vi "Convert String Block.vi"(0 "src buffer in":u8[](array[numeric]), 1 "dst buffer in":u8[](array[numeric]), 2 "src buffer offset":u64 format="%d bytes", 3 "dst buffer offset":u64 format="%d bytes", 4 "channel count":u64, 5 "error in (no error)":errorcluster, 6 "dst data type":T1, 8 "src data type":T1, 10 "dst byte order":T2(ring), 12 "src byte order":T2(ring)) -> (14 "src buffer out":u8[](array[numeric]), 15 "dst buffer out":u8[](array[numeric]), 19 "error out":errorcluster)   [LabVIEW 2017, in "String Type Converter.lvlib" / "String Type Converter.lvclass"]
uses:
  String Type Converter.lvclass
  Builds/Data Sharing Framework/Current/Core/DSF Core.lvlibp/Typedefs/DSF Data Type.ctl
  Builds/Data Sharing Framework/Current/Core/DSF Core.lvlibp/Classes/Framework/Framework.lvclass
  Builds/Data Sharing Framework/Current/Core/DSF Core.lvlibp
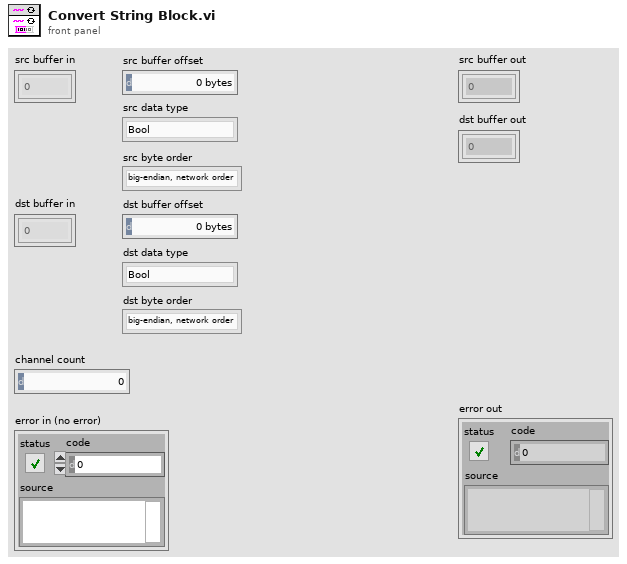
[diagram p1: front panel]
types:
  T1 = typedef "DSF Core.lvlibp/DSF Data Type.ctl" = enum8{"Bool", "SGL", "DBL", "I8", "I16", "I32", "I64", "U8", "U16", "U32", "U64"}
  T2 = enum16{"big-endian, network order", "native, host order", "little-endian"}
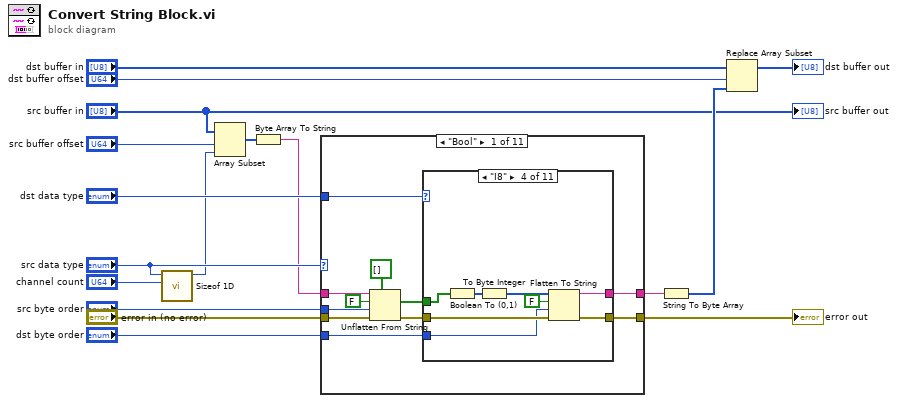
[diagram p0: block diagram]
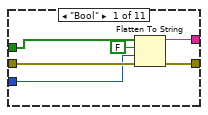
[diagram p2: hidden frame]
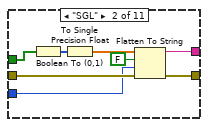
[diagram p3: hidden frame]
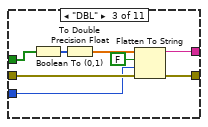
[diagram p4: hidden frame]
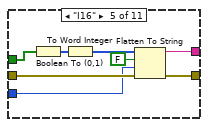
[diagram p5: hidden frame]
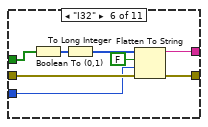
[diagram p6: hidden frame]
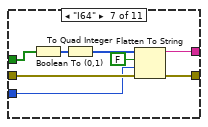
[diagram p7: hidden frame]
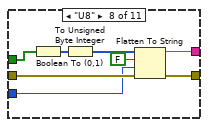
[diagram p8: hidden frame]
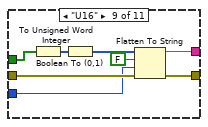
[diagram p9: hidden frame]
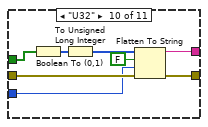
[diagram p10: hidden frame]
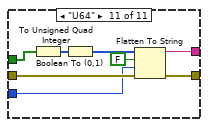
[diagram p11: hidden frame]
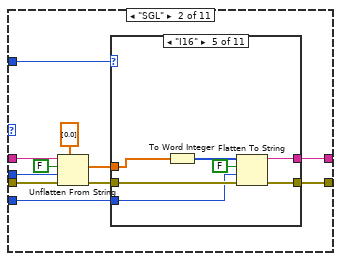
[diagram p12: hidden frame]
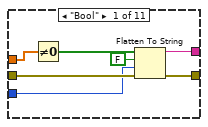
[diagram p13: hidden frame]
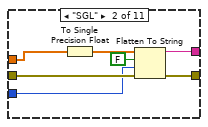
[diagram p14: hidden frame]
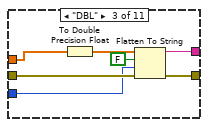
[diagram p15: hidden frame]
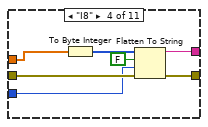
[diagram p16: hidden frame]
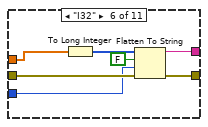
[diagram p17: hidden frame]
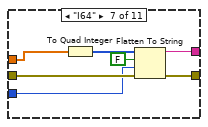
[diagram p18: hidden frame]
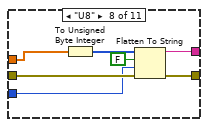
[diagram p19: hidden frame]
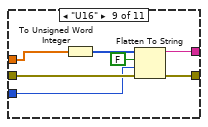
[diagram p20: hidden frame]
diagram:
  n1 = call "Sizeof 1D.vi"("count"="channel count", "data type"="src data type") -> ("size in bytes"=w3:u64)  [unwired: 9 in]
  n2 = Array Subset(array="src buffer in", index="src buffer offset", length=w3) -> (w2:u8[])
  n3 = Byte Array To String(unsigned byte array=w2) -> (string=w1:string)
  n4 = case shown="\"Bool\"" "src data type" {
    tunnel: w1 -> [w26 w123 w211 w299 w387 w475 w563 w651 w739 w827 w915]
    tunnel: "error in (no error)" -> [w25 w122 w210 w298 w386 w474 w562 w650 w738 w826 w914]
    tunnel: "dst data type" -> [w24 w121 w209 w297 w385 w473 w561 w649 w737 w825 w913]
    tunnel: [w21 w118 w206 w294 w382 w470 w558 w646 w734 w822 w910] -> w16
    tunnel: [w20 w117 w205 w293 w381 w469 w557 w645 w733 w821 w909] -> w10
    tunnel: "src byte order" -> [w19 w116 w204 w292 w380 w468 w556 w644 w732 w820 w908]
    tunnel: "dst byte order" -> [w18 w115 w203 w291 w379 w467 w555 w643 w731 w819 w907]
    frame "Bool" {
      n5 = Unflatten From String(type=bool[] [], binary string=w26, data includes array or string size? (T)=FALSE, byte order (0:big-endian, network order)=w19, error in (no error)=w25) -> (value=w23:bool[], error out=w22:errorcluster)  [unwired: 1 out]
      n6 = case shown="\"I8\"" w24 {
        tunnel: w23 -> [w34 w42 w50 w58 w66 w74 w82 w90 w98 w106 w114]
        tunnel: w22 -> [w33 w41 w49 w57 w65 w73 w81 w89 w97 w105 w113]
        tunnel: [w32 w40 w48 w56 w64 w72 w80 w88 w96 w104 w112] -> w21
        tunnel: [w31 w39 w47 w55 w63 w71 w79 w87 w95 w103 w111] -> w20
        tunnel: w18 -> [w30 w38 w46 w54 w62 w70 w78 w86 w94 w102 w110]
        frame "Bool" {
          n7 = Flatten To String(anything=w34, prepend array or string size? (T)=FALSE, byte order (0:big-endian, network order)=w30, error in (no error)=w33) -> (data string=w31:string, error out=w32:errorcluster)  [unwired: 1 out]
        }
        frame "SGL" {
          n8 = Boolean To (0,1)(Boolean=w42) -> (0, 1=w35:i16[])
          n9 = To Single Precision Float(number=w35) -> (single precision float=w36:sgl[])
          n10 = Flatten To String(anything=w36, prepend array or string size? (T)=FALSE, byte order (0:big-endian, network order)=w38, error in (no error)=w41) -> (data string=w39:string, error out=w40:errorcluster)  [unwired: 1 out]
        }
        frame "DBL" {
          n11 = Boolean To (0,1)(Boolean=w50) -> (0, 1=w43:i16[])
          n12 = To Double Precision Float(number=w43) -> (double precision float=w44:dbl[])
          n13 = Flatten To String(anything=w44, prepend array or string size? (T)=FALSE, byte order (0:big-endian, network order)=w46, error in (no error)=w49) -> (data string=w47:string, error out=w48:errorcluster)  [unwired: 1 out]
        }
        frame "I8" {
          n14 = Boolean To (0,1)(Boolean=w58) -> (0, 1=w51:i16[])
          n15 = To Byte Integer(number=w51) -> (8bit integer=w52:i8[])
          n16 = Flatten To String(anything=w52, prepend array or string size? (T)=FALSE, byte order (0:big-endian, network order)=w54, error in (no error)=w57) -> (data string=w55:string, error out=w56:errorcluster)  [unwired: 1 out]
        }
        frame "I16" {
          n17 = Boolean To (0,1)(Boolean=w66) -> (0, 1=w59:i16[])
          n18 = To Word Integer(number=w59) -> (16bit integer=w60:i16[])
          n19 = Flatten To String(anything=w60, prepend array or string size? (T)=FALSE, byte order (0:big-endian, network order)=w62, error in (no error)=w65) -> (data string=w63:string, error out=w64:errorcluster)  [unwired: 1 out]
        }
        frame "I32" {
          n20 = Boolean To (0,1)(Boolean=w74) -> (0, 1=w67:i16[])
          n21 = To Long Integer(number=w67) -> (32bit integer=w68:i32[])
          n22 = Flatten To String(anything=w68, prepend array or string size? (T)=FALSE, byte order (0:big-endian, network order)=w70, error in (no error)=w73) -> (data string=w71:string, error out=w72:errorcluster)  [unwired: 1 out]
        }
        frame "I64" {
          n23 = Boolean To (0,1)(Boolean=w82) -> (0, 1=w75:i16[])
          n24 = To Quad Integer(1:w75) -> (0:w76:i64[])
          n25 = Flatten To String(anything=w76, prepend array or string size? (T)=FALSE, byte order (0:big-endian, network order)=w78, error in (no error)=w81) -> (data string=w79:string, error out=w80:errorcluster)  [unwired: 1 out]
        }
        frame "U8" {
          n26 = Boolean To (0,1)(Boolean=w90) -> (0, 1=w83:i16[])
          n27 = To Unsigned Byte Integer(number=w83) -> (unsigned 8bit integer=w84:u8[])
          n28 = Flatten To String(anything=w84, prepend array or string size? (T)=FALSE, byte order (0:big-endian, network order)=w86, error in (no error)=w89) -> (data string=w87:string, error out=w88:errorcluster)  [unwired: 1 out]
        }
        frame "U16" {
          n29 = Boolean To (0,1)(Boolean=w98) -> (0, 1=w91:i16[])
          n30 = To Unsigned Word Integer(number=w91) -> (unsigned 16bit integer=w92:u16[])
          n31 = Flatten To String(anything=w92, prepend array or string size? (T)=FALSE, byte order (0:big-endian, network order)=w94, error in (no error)=w97) -> (data string=w95:string, error out=w96:errorcluster)  [unwired: 1 out]
        }
        frame "U32" {
          n32 = Boolean To (0,1)(Boolean=w106) -> (0, 1=w99:i16[])
          n33 = To Unsigned Long Integer(number=w99) -> (unsigned 32bit integer=w100:u32[])
          n34 = Flatten To String(anything=w100, prepend array or string size? (T)=FALSE, byte order (0:big-endian, network order)=w102, error in (no error)=w105) -> (data string=w103:string, error out=w104:errorcluster)  [unwired: 1 out]
        }
        frame "U64" {
          n35 = Boolean To (0,1)(Boolean=w114) -> (0, 1=w107:i16[])
          n36 = To Unsigned Quad Integer(1:w107) -> (0:w108:u64[])
          n37 = Flatten To String(anything=w108, prepend array or string size? (T)=FALSE, byte order (0:big-endian, network order)=w110, error in (no error)=w113) -> (data string=w111:string, error out=w112:errorcluster)  [unwired: 1 out]
        }
      }
    }
    frame "SGL" {
      n38 = Unflatten From String(type=sgl[] [0.0], binary string=w123, data includes array or string size? (T)=FALSE, byte order (0:big-endian, network order)=w116, error in (no error)=w122) -> (value=w120:sgl[], error out=w119:errorcluster)  [unwired: 1 out]
      n39 = case shown="\"I16\"" w121 {
        tunnel: w120 -> [w127 w134 w141 w148 w155 w162 w169 w176 w183 w190 w197]
        tunnel: w119 -> [w132 w139 w146 w153 w160 w167 w174 w181 w188 w195 w202]
        tunnel: [w131 w138 w145 w152 w159 w166 w173 w180 w187 w194 w201] -> w118
        tunnel: [w130 w137 w144 w151 w158 w165 w172 w179 w186 w193 w200] -> w117
        tunnel: w115 -> [w129 w136 w143 w150 w157 w164 w171 w178 w185 w192 w199]
        frame "Bool" {
          n40 = Not Equal To 0?(x=w127) -> (x != 0?=w126:bool[])
          n41 = Flatten To String(anything=w126, prepend array or string size? (T)=FALSE, byte order (0:big-endian, network order)=w129, error in (no error)=w132) -> (data string=w130:string, error out=w131:errorcluster)  [unwired: 1 out]
        }
        frame "SGL" {
          n42 = To Single Precision Float(number=w134) -> (single precision float=w133:sgl[])
          n43 = Flatten To String(anything=w133, prepend array or string size? (T)=FALSE, byte order (0:big-endian, network order)=w136, error in (no error)=w139) -> (data string=w137:string, error out=w138:errorcluster)  [unwired: 1 out]
        }
        frame "DBL" {
          n44 = To Double Precision Float(number=w141) -> (double precision float=w140:dbl[])
          n45 = Flatten To String(anything=w140, prepend array or string size? (T)=FALSE, byte order (0:big-endian, network order)=w143, error in (no error)=w146) -> (data string=w144:string, error out=w145:errorcluster)  [unwired: 1 out]
        }
        frame "I8" {
          n46 = To Byte Integer(number=w148) -> (8bit integer=w147:i8[])
          n47 = Flatten To String(anything=w147, prepend array or string size? (T)=FALSE, byte order (0:big-endian, network order)=w150, error in (no error)=w153) -> (data string=w151:string, error out=w152:errorcluster)  [unwired: 1 out]
        }
        frame "I16" {
          n48 = To Word Integer(number=w155) -> (16bit integer=w154:i16[])
          n49 = Flatten To String(anything=w154, prepend array or string size? (T)=FALSE, byte order (0:big-endian, network order)=w157, error in (no error)=w160) -> (data string=w158:string, error out=w159:errorcluster)  [unwired: 1 out]
        }
        frame "I32" {
          n50 = To Long Integer(number=w162) -> (32bit integer=w161:i32[])
          n51 = Flatten To String(anything=w161, prepend array or string size? (T)=FALSE, byte order (0:big-endian, network order)=w164, error in (no error)=w167) -> (data string=w165:string, error out=w166:errorcluster)  [unwired: 1 out]
        }
        frame "I64" {
          n52 = To Quad Integer(1:w169) -> (0:w168:i64[])
          n53 = Flatten To String(anything=w168, prepend array or string size? (T)=FALSE, byte order (0:big-endian, network order)=w171, error in (no error)=w174) -> (data string=w172:string, error out=w173:errorcluster)  [unwired: 1 out]
        }
        frame "U8" {
          n54 = To Unsigned Byte Integer(number=w176) -> (unsigned 8bit integer=w175:u8[])
          n55 = Flatten To String(anything=w175, prepend array or string size? (T)=FALSE, byte order (0:big-endian, network order)=w178, error in (no error)=w181) -> (data string=w179:string, error out=w180:errorcluster)  [unwired: 1 out]
        }
        frame "U16" {
          n56 = To Unsigned Word Integer(number=w183) -> (unsigned 16bit integer=w182:u16[])
          n57 = Flatten To String(anything=w182, prepend array or string size? (T)=FALSE, byte order (0:big-endian, network order)=w185, error in (no error)=w188) -> (data string=w186:string, error out=w187:errorcluster)  [unwired: 1 out]
        }
        frame "U32" {
          n58 = To Unsigned Long Integer(number=w190) -> (unsigned 32bit integer=w189:u32[])
          n59 = Flatten To String(anything=w189, prepend array or string size? (T)=FALSE, byte order (0:big-endian, network order)=w192, error in (no error)=w195) -> (data string=w193:string, error out=w194:errorcluster)  [unwired: 1 out]
        }
        frame "U64" {
          n60 = To Unsigned Quad Integer(1:w197) -> (0:w196:u64[])
          n61 = Flatten To String(anything=w196, prepend array or string size? (T)=FALSE, byte order (0:big-endian, network order)=w199, error in (no error)=w202) -> (data string=w200:string, error out=w201:errorcluster)  [unwired: 1 out]
        }
      }
    }
    frame "DBL" {
      n62 = Unflatten From String(type=dbl[] [0.0], binary string=w211, data includes array or string size? (T)=FALSE, byte order (0:big-endian, network order)=w204, error in (no error)=w210) -> (value=w208:dbl[], error out=w207:errorcluster)  [unwired: 1 out]
      n63 = case shown="\"U64\"" w209 {
        tunnel: w208 -> [w215 w222 w229 w236 w243 w250 w257 w264 w271 w278 w285]
        tunnel: w207 -> [w220 w227 w234 w241 w248 w255 w262 w269 w276 w283 w290]
        tunnel: [w219 w226 w233 w240 w247 w254 w261 w268 w275 w282 w289] -> w206
        tunnel: [w218 w225 w232 w239 w246 w253 w260 w267 w274 w281 w288] -> w205
        tunnel: w203 -> [w217 w224 w231 w238 w245 w252 w259 w266 w273 w280 w287]
        frame "Bool" {
          n64 = Not Equal To 0?(x=w215) -> (x != 0?=w214:bool[])
          n65 = Flatten To String(anything=w214, prepend array or string size? (T)=FALSE, byte order (0:big-endian, network order)=w217, error in (no error)=w220) -> (data string=w218:string, error out=w219:errorcluster)  [unwired: 1 out]
        }
        frame "SGL" {
          n66 = To Single Precision Float(number=w222) -> (single precision float=w221:sgl[])
          n67 = Flatten To String(anything=w221, prepend array or string size? (T)=FALSE, byte order (0:big-endian, network order)=w224, error in (no error)=w227) -> (data string=w225:string, error out=w226:errorcluster)  [unwired: 1 out]
        }
        frame "DBL" {
          n68 = To Double Precision Float(number=w229) -> (double precision float=w228:dbl[])
          n69 = Flatten To String(anything=w228, prepend array or string size? (T)=FALSE, byte order (0:big-endian, network order)=w231, error in (no error)=w234) -> (data string=w232:string, error out=w233:errorcluster)  [unwired: 1 out]
        }
        frame "I8" {
          n70 = To Byte Integer(number=w236) -> (8bit integer=w235:i8[])
          n71 = Flatten To String(anything=w235, prepend array or string size? (T)=FALSE, byte order (0:big-endian, network order)=w238, error in (no error)=w241) -> (data string=w239:string, error out=w240:errorcluster)  [unwired: 1 out]
        }
        frame "I16" {
          n72 = To Word Integer(number=w243) -> (16bit integer=w242:i16[])
          n73 = Flatten To String(anything=w242, prepend array or string size? (T)=FALSE, byte order (0:big-endian, network order)=w245, error in (no error)=w248) -> (data string=w246:string, error out=w247:errorcluster)  [unwired: 1 out]
        }
        frame "I32" {
          n74 = To Long Integer(number=w250) -> (32bit integer=w249:i32[])
          n75 = Flatten To String(anything=w249, prepend array or string size? (T)=FALSE, byte order (0:big-endian, network order)=w252, error in (no error)=w255) -> (data string=w253:string, error out=w254:errorcluster)  [unwired: 1 out]
        }
        frame "I64" {
          n76 = To Quad Integer(1:w257) -> (0:w256:i64[])
          n77 = Flatten To String(anything=w256, prepend array or string size? (T)=FALSE, byte order (0:big-endian, network order)=w259, error in (no error)=w262) -> (data string=w260:string, error out=w261:errorcluster)  [unwired: 1 out]
        }
        frame "U8" {
          n78 = To Unsigned Byte Integer(number=w264) -> (unsigned 8bit integer=w263:u8[])
          n79 = Flatten To String(anything=w263, prepend array or string size? (T)=FALSE, byte order (0:big-endian, network order)=w266, error in (no error)=w269) -> (data string=w267:string, error out=w268:errorcluster)  [unwired: 1 out]
        }
        frame "U16" {
          n80 = To Unsigned Word Integer(number=w271) -> (unsigned 16bit integer=w270:u16[])
          n81 = Flatten To String(anything=w270, prepend array or string size? (T)=FALSE, byte order (0:big-endian, network order)=w273, error in (no error)=w276) -> (data string=w274:string, error out=w275:errorcluster)  [unwired: 1 out]
        }
        frame "U32" {
          n82 = To Unsigned Long Integer(number=w278) -> (unsigned 32bit integer=w277:u32[])
          n83 = Flatten To String(anything=w277, prepend array or string size? (T)=FALSE, byte order (0:big-endian, network order)=w280, error in (no error)=w283) -> (data string=w281:string, error out=w282:errorcluster)  [unwired: 1 out]
        }
        frame "U64" {
          n84 = To Unsigned Quad Integer(1:w285) -> (0:w284:u64[])
          n85 = Flatten To String(anything=w284, prepend array or string size? (T)=FALSE, byte order (0:big-endian, network order)=w287, error in (no error)=w290) -> (data string=w288:string, error out=w289:errorcluster)  [unwired: 1 out]
        }
      }
    }
    frame "I8" {
      n86 = Unflatten From String(type=i8[] [0], binary string=w299, data includes array or string size? (T)=FALSE, byte order (0:big-endian, network order)=w292, error in (no error)=w298) -> (value=w296:i8[], error out=w295:errorcluster)  [unwired: 1 out]
      n87 = case shown="\"Bool\"" w297 {
        tunnel: w296 -> [w303 w310 w317 w324 w331 w338 w345 w352 w359 w366 w373]
        tunnel: w295 -> [w308 w315 w322 w329 w336 w343 w350 w357 w364 w371 w378]
        tunnel: [w307 w314 w321 w328 w335 w342 w349 w356 w363 w370 w377] -> w294
        tunnel: [w306 w313 w320 w327 w334 w341 w348 w355 w362 w369 w376] -> w293
        tunnel: w291 -> [w305 w312 w319 w326 w333 w340 w347 w354 w361 w368 w375]
        frame "Bool" {
          n88 = Not Equal To 0?(x=w303) -> (x != 0?=w302:bool[])
          n89 = Flatten To String(anything=w302, prepend array or string size? (T)=FALSE, byte order (0:big-endian, network order)=w305, error in (no error)=w308) -> (data string=w306:string, error out=w307:errorcluster)  [unwired: 1 out]
        }
        frame "SGL" {
          n90 = To Single Precision Float(number=w310) -> (single precision float=w309:sgl[])
          n91 = Flatten To String(anything=w309, prepend array or string size? (T)=FALSE, byte order (0:big-endian, network order)=w312, error in (no error)=w315) -> (data string=w313:string, error out=w314:errorcluster)  [unwired: 1 out]
        }
        frame "DBL" {
          n92 = To Double Precision Float(number=w317) -> (double precision float=w316:dbl[])
          n93 = Flatten To String(anything=w316, prepend array or string size? (T)=FALSE, byte order (0:big-endian, network order)=w319, error in (no error)=w322) -> (data string=w320:string, error out=w321:errorcluster)  [unwired: 1 out]
        }
        frame "I8" {
          n94 = To Byte Integer(number=w324) -> (8bit integer=w323:i8[])
          n95 = Flatten To String(anything=w323, prepend array or string size? (T)=FALSE, byte order (0:big-endian, network order)=w326, error in (no error)=w329) -> (data string=w327:string, error out=w328:errorcluster)  [unwired: 1 out]
        }
        frame "I16" {
          n96 = To Word Integer(number=w331) -> (16bit integer=w330:i16[])
          n97 = Flatten To String(anything=w330, prepend array or string size? (T)=FALSE, byte order (0:big-endian, network order)=w333, error in (no error)=w336) -> (data string=w334:string, error out=w335:errorcluster)  [unwired: 1 out]
        }
        frame "I32" {
          n98 = To Long Integer(number=w338) -> (32bit integer=w337:i32[])
          n99 = Flatten To String(anything=w337, prepend array or string size? (T)=FALSE, byte order (0:big-endian, network order)=w340, error in (no error)=w343) -> (data string=w341:string, error out=w342:errorcluster)  [unwired: 1 out]
        }
        frame "I64" {
          n100 = To Quad Integer(1:w345) -> (0:w344:i64[])
          n101 = Flatten To String(anything=w344, prepend array or string size? (T)=FALSE, byte order (0:big-endian, network order)=w347, error in (no error)=w350) -> (data string=w348:string, error out=w349:errorcluster)  [unwired: 1 out]
        }
        frame "U8" {
          n102 = To Unsigned Byte Integer(number=w352) -> (unsigned 8bit integer=w351:u8[])
          n103 = Flatten To String(anything=w351, prepend array or string size? (T)=FALSE, byte order (0:big-endian, network order)=w354, error in (no error)=w357) -> (data string=w355:string, error out=w356:errorcluster)  [unwired: 1 out]
        }
        frame "U16" {
          n104 = To Unsigned Word Integer(number=w359) -> (unsigned 16bit integer=w358:u16[])
          n105 = Flatten To String(anything=w358, prepend array or string size? (T)=FALSE, byte order (0:big-endian, network order)=w361, error in (no error)=w364) -> (data string=w362:string, error out=w363:errorcluster)  [unwired: 1 out]
        }
        frame "U32" {
          n106 = To Unsigned Long Integer(number=w366) -> (unsigned 32bit integer=w365:u32[])
          n107 = Flatten To String(anything=w365, prepend array or string size? (T)=FALSE, byte order (0:big-endian, network order)=w368, error in (no error)=w371) -> (data string=w369:string, error out=w370:errorcluster)  [unwired: 1 out]
        }
        frame "U64" {
          n108 = To Unsigned Quad Integer(1:w373) -> (0:w372:u64[])
          n109 = Flatten To String(anything=w372, prepend array or string size? (T)=FALSE, byte order (0:big-endian, network order)=w375, error in (no error)=w378) -> (data string=w376:string, error out=w377:errorcluster)  [unwired: 1 out]
        }
      }
    }
    frame "I16" {
      n110 = Unflatten From String(type=i16[] [0], binary string=w387, data includes array or string size? (T)=FALSE, byte order (0:big-endian, network order)=w380, error in (no error)=w386) -> (value=w384:i16[], error out=w383:errorcluster)  [unwired: 1 out]
      n111 = case shown="\"Bool\"" w385 {
        tunnel: w384 -> [w391 w398 w405 w412 w419 w426 w433 w440 w447 w454 w461]
        tunnel: w383 -> [w396 w403 w410 w417 w424 w431 w438 w445 w452 w459 w466]
        tunnel: [w395 w402 w409 w416 w423 w430 w437 w444 w451 w458 w465] -> w382
        tunnel: [w394 w401 w408 w415 w422 w429 w436 w443 w450 w457 w464] -> w381
        tunnel: w379 -> [w393 w400 w407 w414 w421 w428 w435 w442 w449 w456 w463]
        frame "Bool" {
          n112 = Not Equal To 0?(x=w391) -> (x != 0?=w390:bool[])
          n113 = Flatten To String(anything=w390, prepend array or string size? (T)=FALSE, byte order (0:big-endian, network order)=w393, error in (no error)=w396) -> (data string=w394:string, error out=w395:errorcluster)  [unwired: 1 out]
        }
        frame "SGL" {
          n114 = To Single Precision Float(number=w398) -> (single precision float=w397:sgl[])
          n115 = Flatten To String(anything=w397, prepend array or string size? (T)=FALSE, byte order (0:big-endian, network order)=w400, error in (no error)=w403) -> (data string=w401:string, error out=w402:errorcluster)  [unwired: 1 out]
        }
        frame "DBL" {
          n116 = To Double Precision Float(number=w405) -> (double precision float=w404:dbl[])
          n117 = Flatten To String(anything=w404, prepend array or string size? (T)=FALSE, byte order (0:big-endian, network order)=w407, error in (no error)=w410) -> (data string=w408:string, error out=w409:errorcluster)  [unwired: 1 out]
        }
        frame "I8" {
          n118 = To Byte Integer(number=w412) -> (8bit integer=w411:i8[])
          n119 = Flatten To String(anything=w411, prepend array or string size? (T)=FALSE, byte order (0:big-endian, network order)=w414, error in (no error)=w417) -> (data string=w415:string, error out=w416:errorcluster)  [unwired: 1 out]
        }
        frame "I16" {
          n120 = To Word Integer(number=w419) -> (16bit integer=w418:i16[])
          n121 = Flatten To String(anything=w418, prepend array or string size? (T)=FALSE, byte order (0:big-endian, network order)=w421, error in (no error)=w424) -> (data string=w422:string, error out=w423:errorcluster)  [unwired: 1 out]
        }
        frame "I32" {
          n122 = To Long Integer(number=w426) -> (32bit integer=w425:i32[])
          n123 = Flatten To String(anything=w425, prepend array or string size? (T)=FALSE, byte order (0:big-endian, network order)=w428, error in (no error)=w431) -> (data string=w429:string, error out=w430:errorcluster)  [unwired: 1 out]
        }
        frame "I64" {
          n124 = To Quad Integer(1:w433) -> (0:w432:i64[])
          n125 = Flatten To String(anything=w432, prepend array or string size? (T)=FALSE, byte order (0:big-endian, network order)=w435, error in (no error)=w438) -> (data string=w436:string, error out=w437:errorcluster)  [unwired: 1 out]
        }
        frame "U8" {
          n126 = To Unsigned Byte Integer(number=w440) -> (unsigned 8bit integer=w439:u8[])
          n127 = Flatten To String(anything=w439, prepend array or string size? (T)=FALSE, byte order (0:big-endian, network order)=w442, error in (no error)=w445) -> (data string=w443:string, error out=w444:errorcluster)  [unwired: 1 out]
        }
        frame "U16" {
          n128 = To Unsigned Word Integer(number=w447) -> (unsigned 16bit integer=w446:u16[])
          n129 = Flatten To String(anything=w446, prepend array or string size? (T)=FALSE, byte order (0:big-endian, network order)=w449, error in (no error)=w452) -> (data string=w450:string, error out=w451:errorcluster)  [unwired: 1 out]
        }
        frame "U32" {
          n130 = To Unsigned Long Integer(number=w454) -> (unsigned 32bit integer=w453:u32[])
          n131 = Flatten To String(anything=w453, prepend array or string size? (T)=FALSE, byte order (0:big-endian, network order)=w456, error in (no error)=w459) -> (data string=w457:string, error out=w458:errorcluster)  [unwired: 1 out]
        }
        frame "U64" {
          n132 = To Unsigned Quad Integer(1:w461) -> (0:w460:u64[])
          n133 = Flatten To String(anything=w460, prepend array or string size? (T)=FALSE, byte order (0:big-endian, network order)=w463, error in (no error)=w466) -> (data string=w464:string, error out=w465:errorcluster)  [unwired: 1 out]
        }
      }
    }
    frame "I32" {
      n134 = Unflatten From String(type=i32[] [0], binary string=w475, data includes array or string size? (T)=FALSE, byte order (0:big-endian, network order)=w468, error in (no error)=w474) -> (value=w472:i32[], error out=w471:errorcluster)  [unwired: 1 out]
      n135 = case shown="\"Bool\"" w473 {
        tunnel: w472 -> [w479 w486 w493 w500 w507 w514 w521 w528 w535 w542 w549]
        tunnel: w471 -> [w484 w491 w498 w505 w512 w519 w526 w533 w540 w547 w554]
        tunnel: [w483 w490 w497 w504 w511 w518 w525 w532 w539 w546 w553] -> w470
        tunnel: [w482 w489 w496 w503 w510 w517 w524 w531 w538 w545 w552] -> w469
        tunnel: w467 -> [w481 w488 w495 w502 w509 w516 w523 w530 w537 w544 w551]
        frame "Bool" {
          n136 = Not Equal To 0?(x=w479) -> (x != 0?=w478:bool[])
          n137 = Flatten To String(anything=w478, prepend array or string size? (T)=FALSE, byte order (0:big-endian, network order)=w481, error in (no error)=w484) -> (data string=w482:string, error out=w483:errorcluster)  [unwired: 1 out]
        }
        frame "SGL" {
          n138 = To Single Precision Float(number=w486) -> (single precision float=w485:sgl[])
          n139 = Flatten To String(anything=w485, prepend array or string size? (T)=FALSE, byte order (0:big-endian, network order)=w488, error in (no error)=w491) -> (data string=w489:string, error out=w490:errorcluster)  [unwired: 1 out]
        }
        frame "DBL" {
          n140 = To Double Precision Float(number=w493) -> (double precision float=w492:dbl[])
          n141 = Flatten To String(anything=w492, prepend array or string size? (T)=FALSE, byte order (0:big-endian, network order)=w495, error in (no error)=w498) -> (data string=w496:string, error out=w497:errorcluster)  [unwired: 1 out]
        }
        frame "I8" {
          n142 = To Byte Integer(number=w500) -> (8bit integer=w499:i8[])
          n143 = Flatten To String(anything=w499, prepend array or string size? (T)=FALSE, byte order (0:big-endian, network order)=w502, error in (no error)=w505) -> (data string=w503:string, error out=w504:errorcluster)  [unwired: 1 out]
        }
        frame "I16" {
          n144 = To Word Integer(number=w507) -> (16bit integer=w506:i16[])
          n145 = Flatten To String(anything=w506, prepend array or string size? (T)=FALSE, byte order (0:big-endian, network order)=w509, error in (no error)=w512) -> (data string=w510:string, error out=w511:errorcluster)  [unwired: 1 out]
        }
        frame "I32" {
          n146 = To Long Integer(number=w514) -> (32bit integer=w513:i32[])
          n147 = Flatten To String(anything=w513, prepend array or string size? (T)=FALSE, byte order (0:big-endian, network order)=w516, error in (no error)=w519) -> (data string=w517:string, error out=w518:errorcluster)  [unwired: 1 out]
        }
        frame "I64" {
          n148 = To Quad Integer(1:w521) -> (0:w520:i64[])
          n149 = Flatten To String(anything=w520, prepend array or string size? (T)=FALSE, byte order (0:big-endian, network order)=w523, error in (no error)=w526) -> (data string=w524:string, error out=w525:errorcluster)  [unwired: 1 out]
        }
        frame "U8" {
          n150 = To Unsigned Byte Integer(number=w528) -> (unsigned 8bit integer=w527:u8[])
          n151 = Flatten To String(anything=w527, prepend array or string size? (T)=FALSE, byte order (0:big-endian, network order)=w530, error in (no error)=w533) -> (data string=w531:string, error out=w532:errorcluster)  [unwired: 1 out]
        }
        frame "U16" {
          n152 = To Unsigned Word Integer(number=w535) -> (unsigned 16bit integer=w534:u16[])
          n153 = Flatten To String(anything=w534, prepend array or string size? (T)=FALSE, byte order (0:big-endian, network order)=w537, error in (no error)=w540) -> (data string=w538:string, error out=w539:errorcluster)  [unwired: 1 out]
        }
        frame "U32" {
          n154 = To Unsigned Long Integer(number=w542) -> (unsigned 32bit integer=w541:u32[])
          n155 = Flatten To String(anything=w541, prepend array or string size? (T)=FALSE, byte order (0:big-endian, network order)=w544, error in (no error)=w547) -> (data string=w545:string, error out=w546:errorcluster)  [unwired: 1 out]
        }
        frame "U64" {
          n156 = To Unsigned Quad Integer(1:w549) -> (0:w548:u64[])
          n157 = Flatten To String(anything=w548, prepend array or string size? (T)=FALSE, byte order (0:big-endian, network order)=w551, error in (no error)=w554) -> (data string=w552:string, error out=w553:errorcluster)  [unwired: 1 out]
        }
      }
    }
    frame "I64" {
      n158 = Unflatten From String(type=i64[] [0], binary string=w563, data includes array or string size? (T)=FALSE, byte order (0:big-endian, network order)=w556, error in (no error)=w562) -> (value=w560:i64[], error out=w559:errorcluster)  [unwired: 1 out]
      n159 = case shown="\"Bool\"" w561 {
        tunnel: w560 -> [w567 w574 w581 w588 w595 w602 w609 w616 w623 w630 w637]
        tunnel: w559 -> [w572 w579 w586 w593 w600 w607 w614 w621 w628 w635 w642]
        tunnel: [w571 w578 w585 w592 w599 w606 w613 w620 w627 w634 w641] -> w558
        tunnel: [w570 w577 w584 w591 w598 w605 w612 w619 w626 w633 w640] -> w557
        tunnel: w555 -> [w569 w576 w583 w590 w597 w604 w611 w618 w625 w632 w639]
        frame "Bool" {
          n160 = Not Equal To 0?(x=w567) -> (x != 0?=w566:bool[])
          n161 = Flatten To String(anything=w566, prepend array or string size? (T)=FALSE, byte order (0:big-endian, network order)=w569, error in (no error)=w572) -> (data string=w570:string, error out=w571:errorcluster)  [unwired: 1 out]
        }
        frame "SGL" {
          n162 = To Single Precision Float(number=w574) -> (single precision float=w573:sgl[])
          n163 = Flatten To String(anything=w573, prepend array or string size? (T)=FALSE, byte order (0:big-endian, network order)=w576, error in (no error)=w579) -> (data string=w577:string, error out=w578:errorcluster)  [unwired: 1 out]
        }
        frame "DBL" {
          n164 = To Double Precision Float(number=w581) -> (double precision float=w580:dbl[])
          n165 = Flatten To String(anything=w580, prepend array or string size? (T)=FALSE, byte order (0:big-endian, network order)=w583, error in (no error)=w586) -> (data string=w584:string, error out=w585:errorcluster)  [unwired: 1 out]
        }
        frame "I8" {
          n166 = To Byte Integer(number=w588) -> (8bit integer=w587:i8[])
          n167 = Flatten To String(anything=w587, prepend array or string size? (T)=FALSE, byte order (0:big-endian, network order)=w590, error in (no error)=w593) -> (data string=w591:string, error out=w592:errorcluster)  [unwired: 1 out]
        }
        frame "I16" {
          n168 = To Word Integer(number=w595) -> (16bit integer=w594:i16[])
          n169 = Flatten To String(anything=w594, prepend array or string size? (T)=FALSE, byte order (0:big-endian, network order)=w597, error in (no error)=w600) -> (data string=w598:string, error out=w599:errorcluster)  [unwired: 1 out]
        }
        frame "I32" {
          n170 = To Long Integer(number=w602) -> (32bit integer=w601:i32[])
          n171 = Flatten To String(anything=w601, prepend array or string size? (T)=FALSE, byte order (0:big-endian, network order)=w604, error in (no error)=w607) -> (data string=w605:string, error out=w606:errorcluster)  [unwired: 1 out]
        }
        frame "I64" {
          n172 = To Quad Integer(1:w609) -> (0:w608:i64[])
          n173 = Flatten To String(anything=w608, prepend array or string size? (T)=FALSE, byte order (0:big-endian, network order)=w611, error in (no error)=w614) -> (data string=w612:string, error out=w613:errorcluster)  [unwired: 1 out]
        }
        frame "U8" {
          n174 = To Unsigned Byte Integer(number=w616) -> (unsigned 8bit integer=w615:u8[])
          n175 = Flatten To String(anything=w615, prepend array or string size? (T)=FALSE, byte order (0:big-endian, network order)=w618, error in (no error)=w621) -> (data string=w619:string, error out=w620:errorcluster)  [unwired: 1 out]
        }
        frame "U16" {
          n176 = To Unsigned Word Integer(number=w623) -> (unsigned 16bit integer=w622:u16[])
          n177 = Flatten To String(anything=w622, prepend array or string size? (T)=FALSE, byte order (0:big-endian, network order)=w625, error in (no error)=w628) -> (data string=w626:string, error out=w627:errorcluster)  [unwired: 1 out]
        }
        frame "U32" {
          n178 = To Unsigned Long Integer(number=w630) -> (unsigned 32bit integer=w629:u32[])
          n179 = Flatten To String(anything=w629, prepend array or string size? (T)=FALSE, byte order (0:big-endian, network order)=w632, error in (no error)=w635) -> (data string=w633:string, error out=w634:errorcluster)  [unwired: 1 out]
        }
        frame "U64" {
          n180 = To Unsigned Quad Integer(1:w637) -> (0:w636:u64[])
          n181 = Flatten To String(anything=w636, prepend array or string size? (T)=FALSE, byte order (0:big-endian, network order)=w639, error in (no error)=w642) -> (data string=w640:string, error out=w641:errorcluster)  [unwired: 1 out]
        }
      }
    }
    frame "U8" {
      n182 = Unflatten From String(type=u8[] [0], binary string=w651, data includes array or string size? (T)=FALSE, byte order (0:big-endian, network order)=w644, error in (no error)=w650) -> (value=w648:u8[], error out=w647:errorcluster)  [unwired: 1 out]
      n183 = case shown="\"Bool\"" w649 {
        tunnel: w648 -> [w655 w662 w669 w676 w683 w690 w697 w704 w711 w718 w725]
        tunnel: w647 -> [w660 w667 w674 w681 w688 w695 w702 w709 w716 w723 w730]
        tunnel: [w659 w666 w673 w680 w687 w694 w701 w708 w715 w722 w729] -> w646
        tunnel: [w658 w665 w672 w679 w686 w693 w700 w707 w714 w721 w728] -> w645
        tunnel: w643 -> [w657 w664 w671 w678 w685 w692 w699 w706 w713 w720 w727]
        frame "Bool" {
          n184 = Not Equal To 0?(x=w655) -> (x != 0?=w654:bool[])
          n185 = Flatten To String(anything=w654, prepend array or string size? (T)=FALSE, byte order (0:big-endian, network order)=w657, error in (no error)=w660) -> (data string=w658:string, error out=w659:errorcluster)  [unwired: 1 out]
        }
        frame "SGL" {
          n186 = To Single Precision Float(number=w662) -> (single precision float=w661:sgl[])
          n187 = Flatten To String(anything=w661, prepend array or string size? (T)=FALSE, byte order (0:big-endian, network order)=w664, error in (no error)=w667) -> (data string=w665:string, error out=w666:errorcluster)  [unwired: 1 out]
        }
        frame "DBL" {
          n188 = To Double Precision Float(number=w669) -> (double precision float=w668:dbl[])
          n189 = Flatten To String(anything=w668, prepend array or string size? (T)=FALSE, byte order (0:big-endian, network order)=w671, error in (no error)=w674) -> (data string=w672:string, error out=w673:errorcluster)  [unwired: 1 out]
        }
        frame "I8" {
          n190 = To Byte Integer(number=w676) -> (8bit integer=w675:i8[])
          n191 = Flatten To String(anything=w675, prepend array or string size? (T)=FALSE, byte order (0:big-endian, network order)=w678, error in (no error)=w681) -> (data string=w679:string, error out=w680:errorcluster)  [unwired: 1 out]
        }
        frame "I16" {
          n192 = To Word Integer(number=w683) -> (16bit integer=w682:i16[])
          n193 = Flatten To String(anything=w682, prepend array or string size? (T)=FALSE, byte order (0:big-endian, network order)=w685, error in (no error)=w688) -> (data string=w686:string, error out=w687:errorcluster)  [unwired: 1 out]
        }
        frame "I32" {
          n194 = To Long Integer(number=w690) -> (32bit integer=w689:i32[])
          n195 = Flatten To String(anything=w689, prepend array or string size? (T)=FALSE, byte order (0:big-endian, network order)=w692, error in (no error)=w695) -> (data string=w693:string, error out=w694:errorcluster)  [unwired: 1 out]
        }
        frame "I64" {
          n196 = To Quad Integer(1:w697) -> (0:w696:i64[])
          n197 = Flatten To String(anything=w696, prepend array or string size? (T)=FALSE, byte order (0:big-endian, network order)=w699, error in (no error)=w702) -> (data string=w700:string, error out=w701:errorcluster)  [unwired: 1 out]
        }
        frame "U8" {
          n198 = To Unsigned Byte Integer(number=w704) -> (unsigned 8bit integer=w703:u8[])
          n199 = Flatten To String(anything=w703, prepend array or string size? (T)=FALSE, byte order (0:big-endian, network order)=w706, error in (no error)=w709) -> (data string=w707:string, error out=w708:errorcluster)  [unwired: 1 out]
        }
        frame "U16" {
          n200 = To Unsigned Word Integer(number=w711) -> (unsigned 16bit integer=w710:u16[])
          n201 = Flatten To String(anything=w710, prepend array or string size? (T)=FALSE, byte order (0:big-endian, network order)=w713, error in (no error)=w716) -> (data string=w714:string, error out=w715:errorcluster)  [unwired: 1 out]
        }
        frame "U32" {
          n202 = To Unsigned Long Integer(number=w718) -> (unsigned 32bit integer=w717:u32[])
          n203 = Flatten To String(anything=w717, prepend array or string size? (T)=FALSE, byte order (0:big-endian, network order)=w720, error in (no error)=w723) -> (data string=w721:string, error out=w722:errorcluster)  [unwired: 1 out]
        }
        frame "U64" {
          n204 = To Unsigned Quad Integer(1:w725) -> (0:w724:u64[])
          n205 = Flatten To String(anything=w724, prepend array or string size? (T)=FALSE, byte order (0:big-endian, network order)=w727, error in (no error)=w730) -> (data string=w728:string, error out=w729:errorcluster)  [unwired: 1 out]
        }
      }
    }
    frame "U16" {
      n206 = Unflatten From String(type=u16[] [0], binary string=w739, data includes array or string size? (T)=FALSE, byte order (0:big-endian, network order)=w732, error in (no error)=w738) -> (value=w736:u16[], error out=w735:errorcluster)  [unwired: 1 out]
      n207 = case shown="\"Bool\"" w737 {
        tunnel: w736 -> [w743 w750 w757 w764 w771 w778 w785 w792 w799 w806 w813]
        tunnel: w735 -> [w748 w755 w762 w769 w776 w783 w790 w797 w804 w811 w818]
        tunnel: [w747 w754 w761 w768 w775 w782 w789 w796 w803 w810 w817] -> w734
        tunnel: [w746 w753 w760 w767 w774 w781 w788 w795 w802 w809 w816] -> w733
        tunnel: w731 -> [w745 w752 w759 w766 w773 w780 w787 w794 w801 w808 w815]
        frame "Bool" {
          n208 = Not Equal To 0?(x=w743) -> (x != 0?=w742:bool[])
          n209 = Flatten To String(anything=w742, prepend array or string size? (T)=FALSE, byte order (0:big-endian, network order)=w745, error in (no error)=w748) -> (data string=w746:string, error out=w747:errorcluster)  [unwired: 1 out]
        }
        frame "SGL" {
          n210 = To Single Precision Float(number=w750) -> (single precision float=w749:sgl[])
          n211 = Flatten To String(anything=w749, prepend array or string size? (T)=FALSE, byte order (0:big-endian, network order)=w752, error in (no error)=w755) -> (data string=w753:string, error out=w754:errorcluster)  [unwired: 1 out]
        }
        frame "DBL" {
          n212 = To Double Precision Float(number=w757) -> (double precision float=w756:dbl[])
          n213 = Flatten To String(anything=w756, prepend array or string size? (T)=FALSE, byte order (0:big-endian, network order)=w759, error in (no error)=w762) -> (data string=w760:string, error out=w761:errorcluster)  [unwired: 1 out]
        }
        frame "I8" {
          n214 = To Byte Integer(number=w764) -> (8bit integer=w763:i8[])
          n215 = Flatten To String(anything=w763, prepend array or string size? (T)=FALSE, byte order (0:big-endian, network order)=w766, error in (no error)=w769) -> (data string=w767:string, error out=w768:errorcluster)  [unwired: 1 out]
        }
        frame "I16" {
          n216 = To Word Integer(number=w771) -> (16bit integer=w770:i16[])
          n217 = Flatten To String(anything=w770, prepend array or string size? (T)=FALSE, byte order (0:big-endian, network order)=w773, error in (no error)=w776) -> (data string=w774:string, error out=w775:errorcluster)  [unwired: 1 out]
        }
        frame "I32" {
          n218 = To Long Integer(number=w778) -> (32bit integer=w777:i32[])
          n219 = Flatten To String(anything=w777, prepend array or string size? (T)=FALSE, byte order (0:big-endian, network order)=w780, error in (no error)=w783) -> (data string=w781:string, error out=w782:errorcluster)  [unwired: 1 out]
        }
        frame "I64" {
          n220 = To Quad Integer(1:w785) -> (0:w784:i64[])
          n221 = Flatten To String(anything=w784, prepend array or string size? (T)=FALSE, byte order (0:big-endian, network order)=w787, error in (no error)=w790) -> (data string=w788:string, error out=w789:errorcluster)  [unwired: 1 out]
        }
        frame "U8" {
          n222 = To Unsigned Byte Integer(number=w792) -> (unsigned 8bit integer=w791:u8[])
          n223 = Flatten To String(anything=w791, prepend array or string size? (T)=FALSE, byte order (0:big-endian, network order)=w794, error in (no error)=w797) -> (data string=w795:string, error out=w796:errorcluster)  [unwired: 1 out]
        }
        frame "U16" {
          n224 = To Unsigned Word Integer(number=w799) -> (unsigned 16bit integer=w798:u16[])
          n225 = Flatten To String(anything=w798, prepend array or string size? (T)=FALSE, byte order (0:big-endian, network order)=w801, error in (no error)=w804) -> (data string=w802:string, error out=w803:errorcluster)  [unwired: 1 out]
        }
        frame "U32" {
          n226 = To Unsigned Long Integer(number=w806) -> (unsigned 32bit integer=w805:u32[])
          n227 = Flatten To String(anything=w805, prepend array or string size? (T)=FALSE, byte order (0:big-endian, network order)=w808, error in (no error)=w811) -> (data string=w809:string, error out=w810:errorcluster)  [unwired: 1 out]
        }
        frame "U64" {
          n228 = To Unsigned Quad Integer(1:w813) -> (0:w812:u64[])
          n229 = Flatten To String(anything=w812, prepend array or string size? (T)=FALSE, byte order (0:big-endian, network order)=w815, error in (no error)=w818) -> (data string=w816:string, error out=w817:errorcluster)  [unwired: 1 out]
        }
      }
    }
    frame "U32" {
      n230 = Unflatten From String(type=u32[] [0], binary string=w827, data includes array or string size? (T)=FALSE, byte order (0:big-endian, network order)=w820, error in (no error)=w826) -> (value=w824:u32[], error out=w823:errorcluster)  [unwired: 1 out]
      n231 = case shown="\"Bool\"" w825 {
        tunnel: w824 -> [w831 w838 w845 w852 w859 w866 w873 w880 w887 w894 w901]
        tunnel: w823 -> [w836 w843 w850 w857 w864 w871 w878 w885 w892 w899 w906]
        tunnel: [w835 w842 w849 w856 w863 w870 w877 w884 w891 w898 w905] -> w822
        tunnel: [w834 w841 w848 w855 w862 w869 w876 w883 w890 w897 w904] -> w821
        tunnel: w819 -> [w833 w840 w847 w854 w861 w868 w875 w882 w889 w896 w903]
        frame "Bool" {
          n232 = Not Equal To 0?(x=w831) -> (x != 0?=w830:bool[])
          n233 = Flatten To String(anything=w830, prepend array or string size? (T)=FALSE, byte order (0:big-endian, network order)=w833, error in (no error)=w836) -> (data string=w834:string, error out=w835:errorcluster)  [unwired: 1 out]
        }
        frame "SGL" {
          n234 = To Single Precision Float(number=w838) -> (single precision float=w837:sgl[])
          n235 = Flatten To String(anything=w837, prepend array or string size? (T)=FALSE, byte order (0:big-endian, network order)=w840, error in (no error)=w843) -> (data string=w841:string, error out=w842:errorcluster)  [unwired: 1 out]
        }
        frame "DBL" {
          n236 = To Double Precision Float(number=w845) -> (double precision float=w844:dbl[])
          n237 = Flatten To String(anything=w844, prepend array or string size? (T)=FALSE, byte order (0:big-endian, network order)=w847, error in (no error)=w850) -> (data string=w848:string, error out=w849:errorcluster)  [unwired: 1 out]
        }
        frame "I8" {
          n238 = To Byte Integer(number=w852) -> (8bit integer=w851:i8[])
          n239 = Flatten To String(anything=w851, prepend array or string size? (T)=FALSE, byte order (0:big-endian, network order)=w854, error in (no error)=w857) -> (data string=w855:string, error out=w856:errorcluster)  [unwired: 1 out]
        }
        frame "I16" {
          n240 = To Word Integer(number=w859) -> (16bit integer=w858:i16[])
          n241 = Flatten To String(anything=w858, prepend array or string size? (T)=FALSE, byte order (0:big-endian, network order)=w861, error in (no error)=w864) -> (data string=w862:string, error out=w863:errorcluster)  [unwired: 1 out]
        }
        frame "I32" {
          n242 = To Long Integer(number=w866) -> (32bit integer=w865:i32[])
          n243 = Flatten To String(anything=w865, prepend array or string size? (T)=FALSE, byte order (0:big-endian, network order)=w868, error in (no error)=w871) -> (data string=w869:string, error out=w870:errorcluster)  [unwired: 1 out]
        }
        frame "I64" {
          n244 = To Quad Integer(1:w873) -> (0:w872:i64[])
          n245 = Flatten To String(anything=w872, prepend array or string size? (T)=FALSE, byte order (0:big-endian, network order)=w875, error in (no error)=w878) -> (data string=w876:string, error out=w877:errorcluster)  [unwired: 1 out]
        }
        frame "U8" {
          n246 = To Unsigned Byte Integer(number=w880) -> (unsigned 8bit integer=w879:u8[])
          n247 = Flatten To String(anything=w879, prepend array or string size? (T)=FALSE, byte order (0:big-endian, network order)=w882, error in (no error)=w885) -> (data string=w883:string, error out=w884:errorcluster)  [unwired: 1 out]
        }
        frame "U16" {
          n248 = To Unsigned Word Integer(number=w887) -> (unsigned 16bit integer=w886:u16[])
          n249 = Flatten To String(anything=w886, prepend array or string size? (T)=FALSE, byte order (0:big-endian, network order)=w889, error in (no error)=w892) -> (data string=w890:string, error out=w891:errorcluster)  [unwired: 1 out]
        }
        frame "U32" {
          n250 = To Unsigned Long Integer(number=w894) -> (unsigned 32bit integer=w893:u32[])
          n251 = Flatten To String(anything=w893, prepend array or string size? (T)=FALSE, byte order (0:big-endian, network order)=w896, error in (no error)=w899) -> (data string=w897:string, error out=w898:errorcluster)  [unwired: 1 out]
        }
        frame "U64" {
          n252 = To Unsigned Quad Integer(1:w901) -> (0:w900:u64[])
          n253 = Flatten To String(anything=w900, prepend array or string size? (T)=FALSE, byte order (0:big-endian, network order)=w903, error in (no error)=w906) -> (data string=w904:string, error out=w905:errorcluster)  [unwired: 1 out]
        }
      }
    }
    frame "U64" {
      n254 = Unflatten From String(type=u64[] [0], binary string=w915, data includes array or string size? (T)=FALSE, byte order (0:big-endian, network order)=w908, error in (no error)=w914) -> (value=w912:u64[], error out=w911:errorcluster)  [unwired: 1 out]
      n255 = case shown="\"Bool\"" w913 {
        tunnel: w912 -> [w919 w926 w933 w940 w947 w954 w961 w968 w975 w982 w989]
        tunnel: w911 -> [w924 w931 w938 w945 w952 w959 w966 w973 w980 w987 w994]
        tunnel: [w923 w930 w937 w944 w951 w958 w965 w972 w979 w986 w993] -> w910
        tunnel: [w922 w929 w936 w943 w950 w957 w964 w971 w978 w985 w992] -> w909
        tunnel: w907 -> [w921 w928 w935 w942 w949 w956 w963 w970 w977 w984 w991]
        frame "Bool" {
          n256 = Not Equal To 0?(x=w919) -> (x != 0?=w918:bool[])
          n257 = Flatten To String(anything=w918, prepend array or string size? (T)=FALSE, byte order (0:big-endian, network order)=w921, error in (no error)=w924) -> (data string=w922:string, error out=w923:errorcluster)  [unwired: 1 out]
        }
        frame "SGL" {
          n258 = To Single Precision Float(number=w926) -> (single precision float=w925:sgl[])
          n259 = Flatten To String(anything=w925, prepend array or string size? (T)=FALSE, byte order (0:big-endian, network order)=w928, error in (no error)=w931) -> (data string=w929:string, error out=w930:errorcluster)  [unwired: 1 out]
        }
        frame "DBL" {
          n260 = To Double Precision Float(number=w933) -> (double precision float=w932:dbl[])
          n261 = Flatten To String(anything=w932, prepend array or string size? (T)=FALSE, byte order (0:big-endian, network order)=w935, error in (no error)=w938) -> (data string=w936:string, error out=w937:errorcluster)  [unwired: 1 out]
        }
        frame "I8" {
          n262 = To Byte Integer(number=w940) -> (8bit integer=w939:i8[])
          n263 = Flatten To String(anything=w939, prepend array or string size? (T)=FALSE, byte order (0:big-endian, network order)=w942, error in (no error)=w945) -> (data string=w943:string, error out=w944:errorcluster)  [unwired: 1 out]
        }
        frame "I16" {
          n264 = To Word Integer(number=w947) -> (16bit integer=w946:i16[])
          n265 = Flatten To String(anything=w946, prepend array or string size? (T)=FALSE, byte order (0:big-endian, network order)=w949, error in (no error)=w952) -> (data string=w950:string, error out=w951:errorcluster)  [unwired: 1 out]
        }
        frame "I32" {
          n266 = To Long Integer(number=w954) -> (32bit integer=w953:i32[])
          n267 = Flatten To String(anything=w953, prepend array or string size? (T)=FALSE, byte order (0:big-endian, network order)=w956, error in (no error)=w959) -> (data string=w957:string, error out=w958:errorcluster)  [unwired: 1 out]
        }
        frame "I64" {
          n268 = To Quad Integer(1:w961) -> (0:w960:i64[])
          n269 = Flatten To String(anything=w960, prepend array or string size? (T)=FALSE, byte order (0:big-endian, network order)=w963, error in (no error)=w966) -> (data string=w964:string, error out=w965:errorcluster)  [unwired: 1 out]
        }
        frame "U8" {
          n270 = To Unsigned Byte Integer(number=w968) -> (unsigned 8bit integer=w967:u8[])
          n271 = Flatten To String(anything=w967, prepend array or string size? (T)=FALSE, byte order (0:big-endian, network order)=w970, error in (no error)=w973) -> (data string=w971:string, error out=w972:errorcluster)  [unwired: 1 out]
        }
        frame "U16" {
          n272 = To Unsigned Word Integer(number=w975) -> (unsigned 16bit integer=w974:u16[])
          n273 = Flatten To String(anything=w974, prepend array or string size? (T)=FALSE, byte order (0:big-endian, network order)=w977, error in (no error)=w980) -> (data string=w978:string, error out=w979:errorcluster)  [unwired: 1 out]
        }
        frame "U32" {
          n274 = To Unsigned Long Integer(number=w982) -> (unsigned 32bit integer=w981:u32[])
          n275 = Flatten To String(anything=w981, prepend array or string size? (T)=FALSE, byte order (0:big-endian, network order)=w984, error in (no error)=w987) -> (data string=w985:string, error out=w986:errorcluster)  [unwired: 1 out]
        }
        frame "U64" {
          n276 = To Unsigned Quad Integer(1:w989) -> (0:w988:u64[])
          n277 = Flatten To String(anything=w988, prepend array or string size? (T)=FALSE, byte order (0:big-endian, network order)=w991, error in (no error)=w994) -> (data string=w992:string, error out=w993:errorcluster)  [unwired: 1 out]
        }
      }
    }
  }
  "error out" <- w16
  n278 = String To Byte Array(string=w10) -> (unsigned byte array=w9:u8[])
  n279 = Replace Array Subset(array="dst buffer in", new element=w9, index="dst buffer offset") -> (→"dst buffer out":u8[])
  "src buffer out" <- "src buffer in"
